vi "Set Position.vi"(8 "error in":errorcluster, 9 "Datum":T1, 10 "Target Coordinates":T2, 11 "Flex Subpanel in":refnum<class "Flex UI Subpanel.lvclass">) -> (0 "error out":errorcluster, 3 "Flex Subpanel out":refnum<class "Flex UI Subpanel.lvclass">)   [LabVIEW 2016, in "Flex UI Subpanel.lvclass"]
doc: "Sets the position of the UI.\n\nThe Datum input specifies which part of the VI panel should be sent to those coordinates. For example, the Top-Left (corner) versus the Center point of the panel."
uses:
  Flex UI Subpanel.lvclass
  <vilib>/Utility/miscctls.llb/LVPositionTypeDef.ctl
  Flex UI (Parent)/Enum - Datum.ctl
  Flex UI Subpanel.lvclass/Flex UI Subpanel.ctl
  Flex UI (Parent)/Flex UI.lvclass
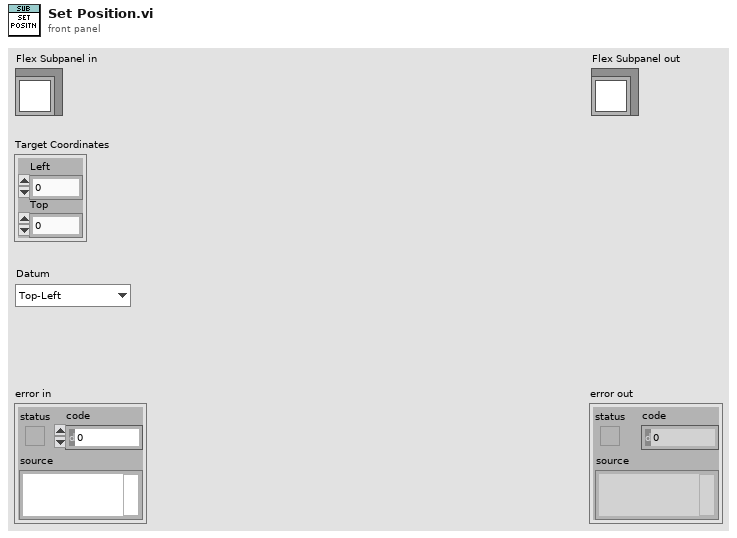
[diagram p1: front panel]
types:
  T1 = typedef "Flex UI.lvclass/Enum - Datum.ctl" = enum16{"Top-Left", "Top-Right", "Bottom-Left", "Bottom-Right", "Center"}
  T2 = typedef "LVPositionTypeDef.ctl" = cluster{"Left":i32, "Top":i32}
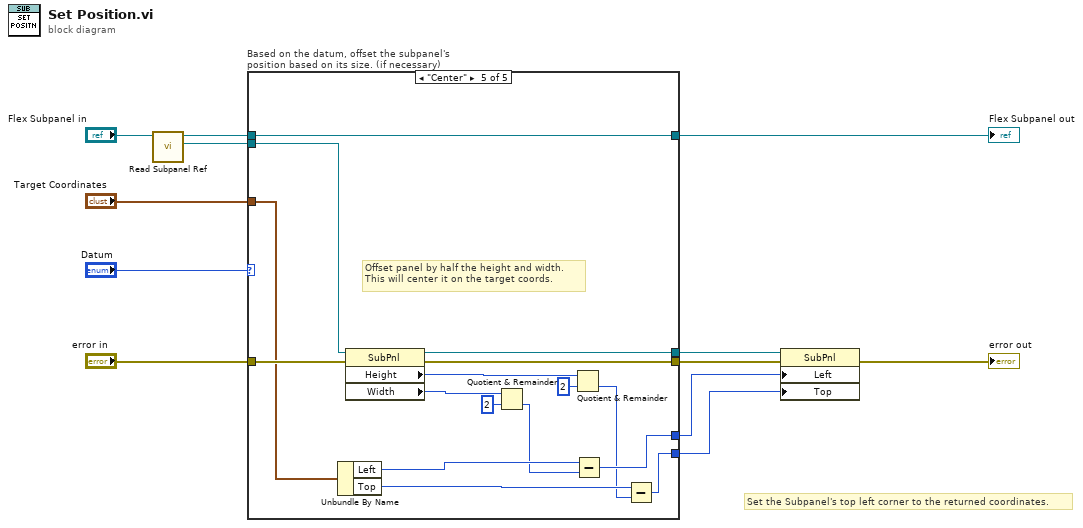
[diagram p0: block diagram]
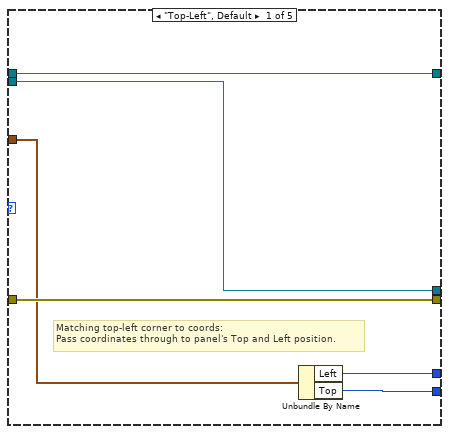
[diagram p2: hidden frame]
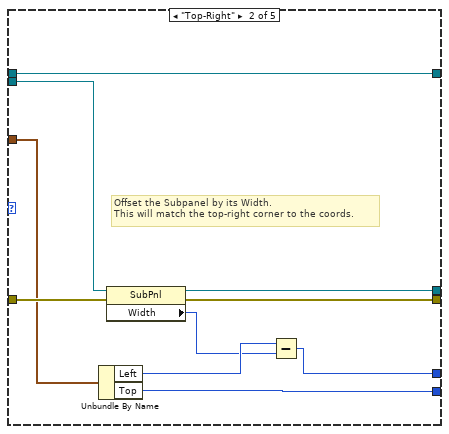
[diagram p3: hidden frame]
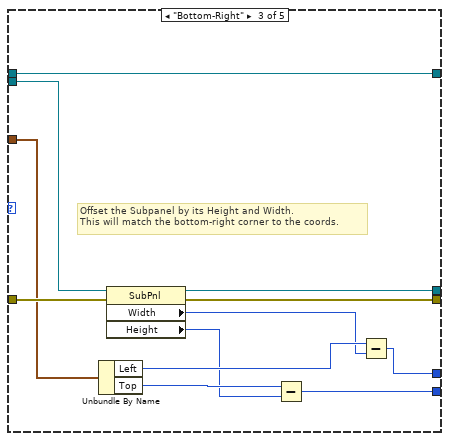
[diagram p4: hidden frame]
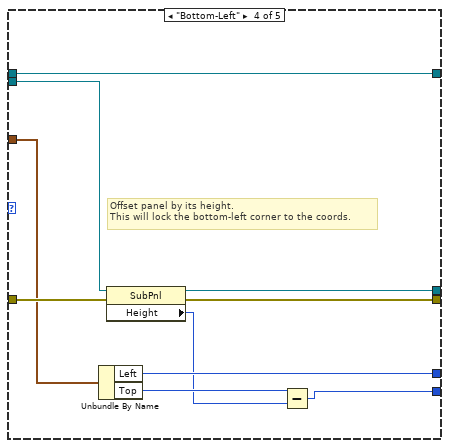
[diagram p5: hidden frame]
diagram:
  # "Set the Subpanel's top left corner to the returned coordinates."
  n1 = call "Read Subpanel Ref.vi"("Flex Subpanel in"="Flex Subpanel in") -> ("Subpanel Ref"=w3:refnum<vi>, "Flex Subpanel out"=w4:refnum<class "Flex UI Subpanel.lvclass">)  [unwired: 9 in]
  n2 = case "Based on the datum, offset the subpanel's position based on its size. (if necessary)" shown="\"Center\"" "Datum" {
    tunnel: [w18 w28 w40 w50 w66] -> w8
    tunnel: w4 -> [w18 w28 w40 w50 w66]
    tunnel: [w17 w24 w37 w47 w63] -> w12
    tunnel: "error in" -> [w17 w27 w39 w49 w65]
    tunnel: "Target Coordinates" -> [w16 w26 w38 w48 w64]
    tunnel: [w15 w21 w34 w46 w59] -> w11
    tunnel: [w14 w25 w32 w43 w61] -> w10
    tunnel: w3 -> [w13 w20 w30 w42 w58]
    tunnel: [w13 w19 w29 w41 w57] -> w1
    frame "Top-Left", Default {
      # "Matching top-left corner to coords:\nPass coordinates through to panel's Top and Left position."
      n3 = Unbundle By Name(w16) -> ("Left"=w15:i32, "Top"=w14:i32)
    }
    frame "Top-Right" {
      # "Offset the Subpanel by its Width.\nThis will match the top-right corner to the coords."
      n4 = Unbundle By Name(w26) -> ("Left"=w23:i32, "Top"=w25:i32)
      n5 = property class="SubPnl"(reference=w20, error in=w27) -> (reference out=w19:refnum<vi>, error out=w24:errorcluster, "Width"=w22:u32)
      n6 = Subtract(x=w23, y=w22) -> (x-y=w21:u32)
    }
    frame "Bottom-Right" {
      # "Offset the Subpanel by its Height and Width.\nThis will match the bottom-right corner to the coords."
      n7 = Unbundle By Name(w38) -> ("Left"=w36:i32, "Top"=w33:i32)
      n8 = property class="SubPnl"(reference=w30, error in=w39) -> (reference out=w29:refnum<vi>, error out=w37:errorcluster, "Width"=w35:u32, "Height"=w31:u32)
      n9 = Subtract(x=w33, y=w31) -> (x-y=w32:u32)
      n10 = Subtract(x=w36, y=w35) -> (x-y=w34:u32)
    }
    frame "Bottom-Left" {
      # "Offset panel by its height.\nThis will lock the bottom-left corner to the coords."
      n11 = Unbundle By Name(w48) -> ("Left"=w46:i32, "Top"=w45:i32)
      n12 = property class="SubPnl"(reference=w42, error in=w49) -> (reference out=w41:refnum<vi>, error out=w47:errorcluster, "Height"=w44:u32)
      n13 = Subtract(x=w45, y=w44) -> (x-y=w43:u32)
    }
    frame "Center" {
      # "Offset panel by half the height and width.\nThis will center it on the target coords."
      n14 = Unbundle By Name(w64) -> ("Left"=w60:i32, "Top"=w62:i32)
      n15 = property class="SubPnl"(reference=w58, error in=w65) -> (reference out=w57:refnum<vi>, error out=w63:errorcluster, "Height"=w55:u32, "Width"=w52:u32)
      n16 = Quotient & Remainder(x=w52, y=u32 2) -> (floor(x/y)=w51:u32)  [unwired: 1 out]
      n17 = Quotient & Remainder(x=w55, y=u32 2) -> (floor(x/y)=w56:u32)  [unwired: 1 out]
      n18 = Subtract(x=w60, y=w51) -> (x-y=w59:u32)
      n19 = Subtract(x=w62, y=w56) -> (x-y=w61:u32)
    }
  }
  "Flex Subpanel out" <- w8
  n20 = property class="SubPnl"(reference=w1, error in=w12, "Left"=w11, "Top"=w10) -> (error out=→"error out":errorcluster)  [unwired: 1 out]
